vi "Fgen Instrument UI.vi"() -> ()   [LabVIEW 2025, in "Fgen.lvlib" / "Fgen Instrument.lvclass"]
doc: "Copyright 2017 National Instruments Corporation\n\nLicensed under the Apache License, Version 2.0 (the \"License\"); you may not use this file except in compliance with the License. You may obtain a copy of the License at http://www.apache.org/licenses/LICENSE-2.0\nUnless required by applicable law or agreed to in writing, software distributed under the License is distributed on an \"AS IS\" BASIS, WITHOUT WARRANTIES OR CONDITIONS OF ANY KIND, either express or implied. See the License for the specific language governing permissions and limitations under the License."
uses:
  Fgen Instrument.lvclass
  Users/Public/Documents/Sandia National Labs/TSS Plugin/CEF.lvlibp/Node/NodeRef.ctl
  Users/Public/Documents/Sandia National Labs/TSS Plugin/CEF.lvlibp/Node/CEF_Node.lvclass
  Users/Public/Documents/Sandia National Labs/TSS Plugin/CEF.lvlibp/Node/mainQref.ctl
  Users/Public/Documents/Sandia National Labs/TSS Plugin/CEF.lvlibp/Node/UserEventRef.ctl
  Users/Public/Documents/Sandia National Labs/TSS Plugin/Abstract Engine.lvlibp/Instrument configuration/Default Instrument.ctl
  Fgen configuration/Fgen Setting.ctl
  C:/Users/Public/Documents/Sandia National Labs/TSS Plugin/CEF.lvlibp/Node/CEF_Node.lvclass
  Fgen Instrument.lvclass/Fgen Instrument.ctl
  Fgen configuration/Fgen configuration.lvclass/Fgen configuration.ctl
  Fgen configuration/Read Fgen Setting.vi
  Fgen configuration/Write Fgen Setting.vi
  <vilib>/Utility/error.llb/Trim Whitespace One-Sided.vi
  Fgen configuration/Fgen configuration.lvclass
  C:/Users/Public/Documents/Sandia National Labs/TSS Plugin/Abstract Engine.lvlibp/Instrument configuration/Instrument configuration.lvclass
  Users/Public/Documents/Sandia National Labs/TSS Plugin/Abstract Engine.lvlibp/Instrument configuration/Read Instrument Setting.vi
  Users/Public/Documents/Sandia National Labs/TSS Plugin/Abstract Engine.lvlibp/Instrument configuration/Write Instrument Setting.vi
  Users/Public/Documents/Sandia National Labs/TSS Plugin/Abstract Engine.lvlibp/Instrument configuration/Instrument configuration.lvclass
panel:
  in  "Fgen":cluster{"Default":T1, "Setting":T2}={"Default"={"Type"="Foundation Bus", "Address"="None", "SW Alias"="None", "Description"="* Type = Class", "Enabled"=TRUE}, "Setting"={"Type"="Arbitrary Waveform", "Output Mode"="Arbitrary Waveform", "Sample Rate"=1000000.0, "Samples"=100000.0, "Gain"=1.0, "Trigger"="Script Trigger", "Impedance"="50", "Offset"=0.0}} {"Setting"."Samples" format="%#_6p"; "Setting"."Sample Rate" format="%#_6p"}
  in  "user event":T3
  in  "main queue":T4
  in  "node ref":T5
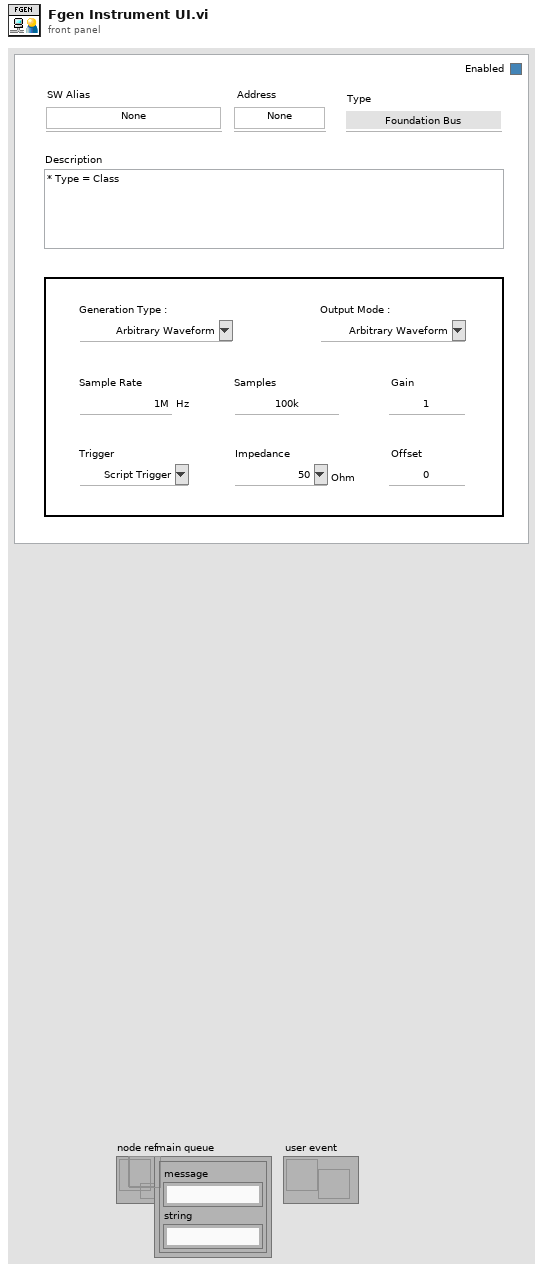
[diagram p1: front panel]
types:
  T1 = typedef "Abstract Engine.lvlibp/Instrument configuration.lvclass/Default Instrument.ctl" = cluster{"Type":string, "Address":string, "SW Alias":string, "Description":string, "Enabled":bool}
  T2 = typedef "Fgen.lvlib/Fgen configuration.lvclass/Fgen Setting.ctl" = cluster{"Type":string, "Output Mode":string, "Sample Rate":dbl, "Samples":dbl, "Gain":dbl, "Trigger":string, "Impedance":string, "Offset":dbl}
  T3 = typedef "CEF.lvlibp/CEF_Node.lvclass/UserEventRef.ctl" = refnum<user-event>
  T4 = typedef "CEF.lvlibp/CEF_Node.lvclass/mainQref.ctl" = refnum<queue>
  T5 = typedef "CEF.lvlibp/CEF_Node.lvclass/NodeRef.ctl" = refnum<data-value>
  T6 = cluster{"Instrument Setting":T1, "Fgen Setting":T2}
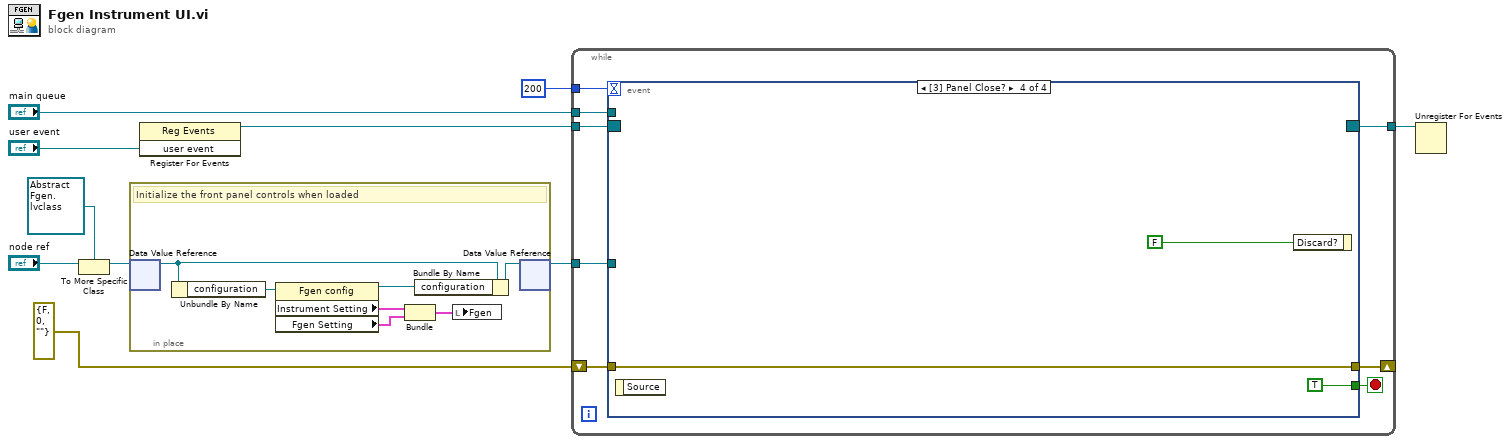
[diagram p0: block diagram]
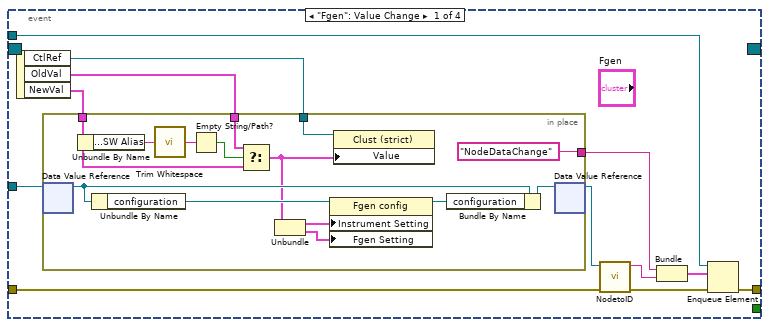
[diagram p2: hidden frame]
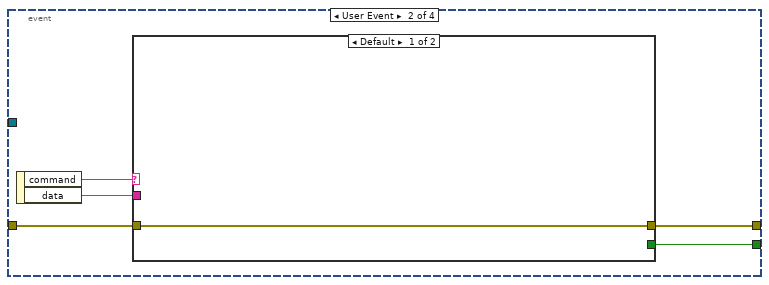
[diagram p3: hidden frame]
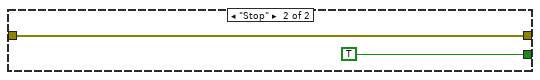
[diagram p4: hidden frame]
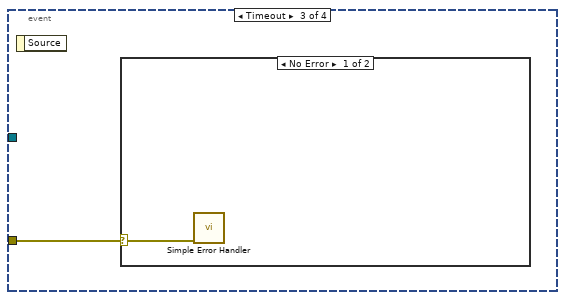
[diagram p5: hidden frame]
diagram:
  n1 = To More Specific Class(target class=refnum<data-value> refnum ("data value reference"), reference="node ref") -> (specific class reference=w6:refnum<data-value>)  [unwired: 1 in, 1 out]
  n2 = in-place {
    # "Initialize the front panel controls when loaded"
    n3 = in-place-dvr #1(w6) -> (w16:refnum<class "Fgen Instrument.lvclass">)  [unwired: 1 out]
    n4 = Unbundle By Name(w16) -> ("configuration"=w17:refnum<class "Fgen configuration.lvclass">)
    n5 = property class="Fgen config"(reference=w17) -> (reference out=w15:refnum<class "Fgen configuration.lvclass">, "Instrument Setting"=w12:T1, "Fgen Setting"=w11:T2)  [unwired: 1 in, 1 out]
    n6 = Bundle("Instrument Setting"=w12, "Fgen Setting"=w11) -> (w13:T6)  [unwired: 1 in]
    n7 = Bundle By Name(cluster=w16, "configuration"=w15) -> (w14:refnum<class "Fgen Instrument.lvclass">)
    n8 = local write "Fgen"(w13) -> ()
    n9 = in-place-dvr #1(w14) -> (w4:refnum<data-value>)  [unwired: 1 out]
  }
  n10 = register-events("user event") -> (reference out=w8:refnum<event-registration>)  [unwired: 2 in, 1 out]
  n11 = while {
    tunnel: "main queue" -> [w24]
    tunnel: w8 -> [w22]
    tunnel: [w21] -> w7
    tunnel: w4 -> [w19]
    shift-right: [w23] -> _
    shift-left: errorcluster {"status"=FALSE, "code"=0, "source"=""} ("error out") -> [w25]
    tunnel: 200 -> [w18]
    stop <- w20 stop-if-true
    n12 = event shown="[3] Panel Close?" {
      selector: w22 -> [_ _ _ _]
      dyn-events: [_ _ _ _] -> w21
      timeout: w18 -> [_ _ _ _]
      tunnel: [w37 w53 _ w63] -> w23
      tunnel: w25 -> [w27 w54 w60 w63]
      tunnel: w24 -> [w36 _ _ _]
      tunnel: w19 -> [w35 _ _ _]
      tunnel: [_ w52 _ TRUE] -> w20
      event "Fgen": Value Change {
        n13 = event-data() -> ("CtlRef"=w31:refnum<vi>, "OldVal"=w32:cluster{"Default":T1, "Setting":T2}, "NewVal"=w33:cluster{"Default":T1, "Setting":T2})  [unwired: 1 in]
        n14 = in-place {
          in-place-border: w33 -> [w46]
          in-place-border: w32 -> [w49]
          in-place-border: w31 -> [w48]
          in-place-border: ["NodeDataChange" ("Message Name")] -> w29
          n15 = in-place-dvr #2(w35) -> (w51:refnum<class "Fgen Instrument.lvclass">)  [unwired: 1 out]
          n16 = Unbundle By Name(w46) -> ("Default.SW Alias"=w47:string)
          n17 = Unbundle By Name(w51) -> ("configuration"=w43:refnum<class "Fgen configuration.lvclass">)
          n18 = call <vilib>:"Trim Whitespace.vi"("string"=w47) -> ("trimmed string"=w44:string)  [unwired: 1 in]
          n19 = Empty String/Path?(string/path=w44) -> (empty?=w45:bool)
          n20 = Select(t=w49, s=w45, f=w46) -> (s? t:f=w41:cluster{"Default":T1, "Setting":T2})
          n21 = Unbundle(w41) -> ("Default"=w40:T1, "Setting"=w39:T2)
          n22 = property class="Fgen config"(reference=w43, "Instrument Setting"=w40, "Fgen Setting"=w39) -> (reference out=w42:refnum<class "Fgen configuration.lvclass">)  [unwired: 1 in, 1 out]
          n23 = property class="Clust (strict)"(reference=w48, "Value"=w41) -> ()  [unwired: 1 in, 2 out]
          n24 = Bundle By Name(cluster=w51, "configuration"=w42) -> (w50:refnum<class "Fgen Instrument.lvclass">)
          n25 = in-place-dvr #2(w50) -> (w34:refnum<data-value>)  [unwired: 1 out]
        }
        n26 = call "NodetoID.vi"("error in"=w27, "node ref"=w34) -> ("error out"=w26:errorcluster, "ID"=w28:string)  [unwired: 8 in]
        n27 = Bundle("Message Name"=w29, "ID"=w28) -> (w30:cluster{"Message Name":string, "ID":string})  [unwired: 1 in]
        n28 = Enqueue Element(queue=w36, element=w30, error in (no error)=w26) -> (error out=w37:errorcluster)  [unwired: 1 in, 2 out]
      }
      event User Event {
        n29 = event-data() -> ("command"=w56:string, "data"=w55:string)  [unwired: 1 in]
        n30 = case shown="Default" w56 {
          tunnel: w55 -> [_ _]
          tunnel: w54 -> [w57 w58]
          tunnel: [w57 w58] -> w53
          tunnel: [_ TRUE] -> w52
          frame Default {
          }
          frame "Stop" {
          }
        }
      }
      event Timeout {
        n31 = event-data() -> ()  [unwired: 1 in, 1 out]
        n32 = case shown="No Error" w60 {
          selector: w60 -> [w61 _]
          frame No Error {
            n33 = call <vilib>:"Simple Error Handler.vi"("error in (no error)"=w61) -> ()  [unwired: 4 in, 5 out]
          }
          frame Error {
          }
        }
      }
      event Panel Close? {
        n34 = event-data() -> ()  [unwired: 1 in, 1 out]
        n35 = event-data("Discard?"=FALSE) -> ()  [unwired: 1 in, 1 out]
      }
    }
  }
  n36 = Unregister For Events(event registration refnum=w7) -> ()  [unwired: 1 in, 1 out]
